vi "WAMP to LV error.vi"(8 "error in (no error)":errorcluster, 9 "Details Index":u32=3, 11 "WAMP Message":T3 {"Message Codes" items=["HELLO"=1, "WELCOME"=2, "ABORT"=3, "GOODBYE"=6, "ERROR"=8, "PUBLISH"=16, "PUBLISHED"=17, "SUBSCRIBE"=32, "SUBSCRIBED"=33, "UNSUBSCRIBE"=34, "UNSUBSCRIBED"=35, "EVENT"=36, "CALL"=48, "RESULT"=59, "REGISTER"=64, "REGISTERED"=65, "UNREGISTER"=66, "UNREGISTERED"=67, "INVOCATION"=68, "YIELD"=70]}) -> (0 "error out":errorcluster, 1 "Wamp Error":T2={"Details"="{}", "ArgumentKw Payload"="{}", "Error?"=FALSE, "Error URI"="", "Arguments Payload"=""}, 3 "Combined Error":T1={"Error?"=FALSE, "WAMP Error"={"Details"="{}", "ArgumentKw Payload"="{}", "Error?"=FALSE, "Error URI"="", "Arguments Payload"=""}, "Error"={"status"=FALSE, "code"=0, "source"=""}})   [LabVIEW 2020, in "wamplv.lvlib" / "WAMP Client.lvclass"]
uses:
  WAMP Client.lvclass
  WAMP Client.lvclass/WAMP Client.ctl
  TypeDef/WAMP Message Codes.ctl
  TypeDef/WAMP Received Message.ctl
  API/TypeDefs/WAMP error.ctl
  API/TypeDefs/Combined error.ctl
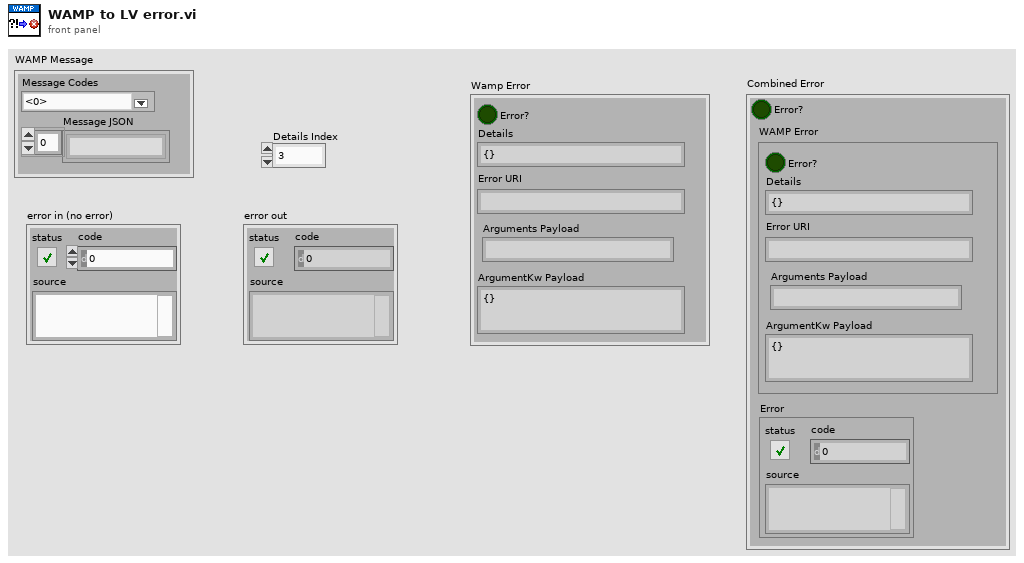
[diagram p1: front panel]
types:
  T1 = typedef "wamplv.lvlib/WAMP Client.lvclass/Combined error.ctl" = cluster{"Error?":bool, "WAMP Error":T2, "Error":errorcluster}
  T2 = typedef "wamplv.lvlib/WAMP Client.lvclass/WAMP error.ctl" = cluster{"Details":string, "ArgumentKw Payload":string, "Error?":bool, "Error URI":string, "Arguments Payload":string}
  T3 = typedef "wamplv.lvlib/WAMP Client.lvclass/WAMP Received Message.ctl" = cluster{"Message JSON":string[], "Message Codes":T4}
  T4 = typedef "wamplv.lvlib/WAMP Client.lvclass/WAMP Message Codes.ctl" = u16
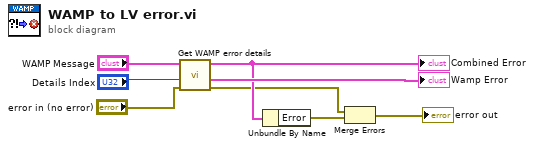
[diagram p0: block diagram]
diagram:
  n1 = call "Get WAMP error details.vi"("error in (no error)"="error in (no error)", "Details Index"="Details Index", "WAMP Message"="WAMP Message") -> ("error out"=w1:errorcluster, "Wamp Error"=→"Wamp Error":T2, "Combined Error"=w4:T1)  [unwired: 6 in]
  "Combined Error" <- w4
  n2 = Unbundle By Name(w4) -> ("Error"=w2:errorcluster)
  n3 = Merge Errors(w1, w2) -> (→"error out":errorcluster)
